vi "Check Time Range.vi"(9 "End":dbl, 10 "Start":dbl, 11 "Time":dbl[](array[numeric])) -> (1 "Incomplete End":dbl, 2 "Incomplete Start":dbl, 3 "Complete Range":bool)   [LabVIEW 2020, in "VolatusHistorian.lvlib" / "Group Buffer DBL.lvclass"]
uses:
  Group Buffer DBL.lvclass
  Group Buffer DBL.lvclass/Group Buffer DBL.ctl
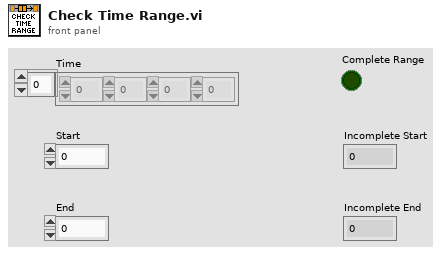
[diagram p1: front panel]
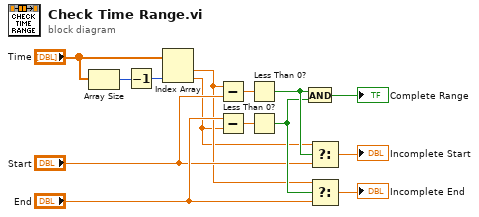
[diagram p0: block diagram]
diagram:
  n1 = Array Size(array="Time") -> (size(s)=w14:i32)
  n2 = Decrement(x=w14) -> (x-1=w13:i32)
  n3 = Index Array(array="Time", index #2=w13) -> (element #1=w3:dbl, element #2=w2:dbl)  [unwired: 1 in]
  n4 = Subtract(x=w3, y="Start") -> (x-y=w12:dbl)
  n5 = Subtract(x="End", y=w2) -> (x-y=w11:dbl)
  n6 = Less Than 0?(x=w12) -> (x < 0?=w9:bool)
  n7 = Less Than 0?(x=w11) -> (x < 0?=w7:bool)
  n8 = And(x=w9, y=w7) -> (x .and. y?=→"Complete Range":bool)
  n9 = Select(t=w2, s=w9, f="Start") -> (s? t:f=→"Incomplete Start":dbl)
  n10 = Select(t=w3, s=w7, f="End") -> (s? t:f=→"Incomplete End":dbl)
